vi "VI Tree.vi"   [LabVIEW 2019]
uses:
  Get Async.lvlib
  <vilib>/httpClient/ClientHandle.ctl
  <vilib>/httpClient/LabVIEWHTTPClient.lvlib
types:
  T1 = typedef "LabVIEWHTTPClient.lvlib/ClientHandle.ctl" = refnum<k1>
  T2 = typedef "HTTP Client Extensions.lvlib/Get Async.lvlib/Refnum Type.ctl" = refnum<k1>
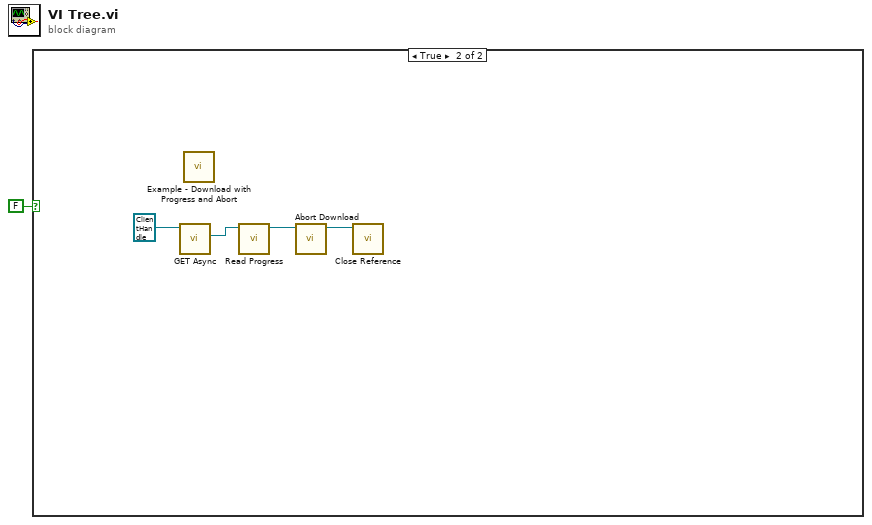
[diagram p0: block diagram]
diagram:
  n1 = case shown="True" FALSE {
    frame False {
    }
    frame True {
      n2 = call "GET Async.vi"("client handle"=T1 refnum) -> ("get async handle"=w5:T2)  [unwired: 7 in, 3 out]
      n3 = call "Example - Download with Progress and Abort.vi"() -> ()  [unwired: 12 in]
      n4 = call "Read Progress.vi"("HTTP GET Async handle"=w5) -> ("HTTP GET Async handle out"=w4:T2)  [unwired: 5 in, 5 out]
      n5 = call "Abort Download.vi"("HTTP GET Async handle"=w4) -> ("HTTP GET Async handle out"=w3:T2)  [unwired: 9 in, 1 out]
      n6 = call "Close Reference.vi"("HTTP GET Async handle"=w3) -> ()  [unwired: 10 in, 1 out]
    }
  }
